vi "Build Table Results.vi"(11 "Table result references":T1) -> (3 "Table values":string[][](array[string]), 5 "Column headers":string[](array[string]))   [LabVIEW 2021, in "Single Tone_Audio DAC.lvlib"]
uses:
  Single Tone_Audio DAC.lvlib
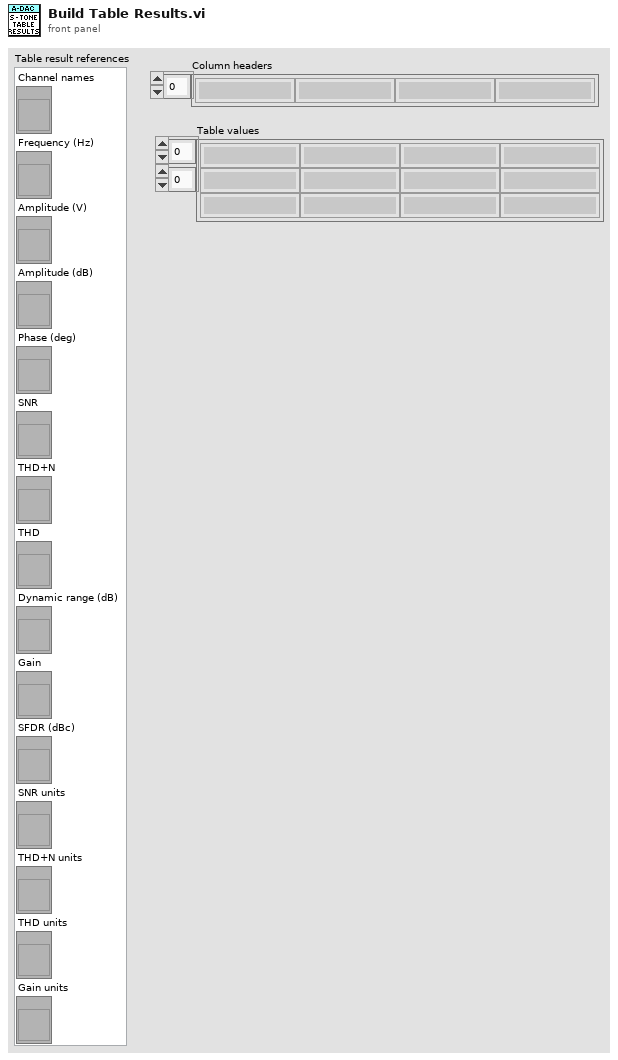
[diagram p1: front panel]
types:
  T1 = cluster{"Channel names":refnum<vi>, "Frequency (Hz)":refnum<vi>, "Amplitude (V)":refnum<vi>, "Amplitude (dB)":refnum<vi>, "Phase (deg)":refnum<vi>, "SNR":refnum<vi>, "THD+N":refnum<vi>, "THD":refnum<vi>, "Dynamic range (dB)":refnum<vi>, "Gain":refnum<vi>, "SFDR (dBc)":refnum<vi>, "SNR units":refnum<vi>, "THD+N units":refnum<vi>, "THD units":refnum<vi>, "Gain units":refnum<vi>}
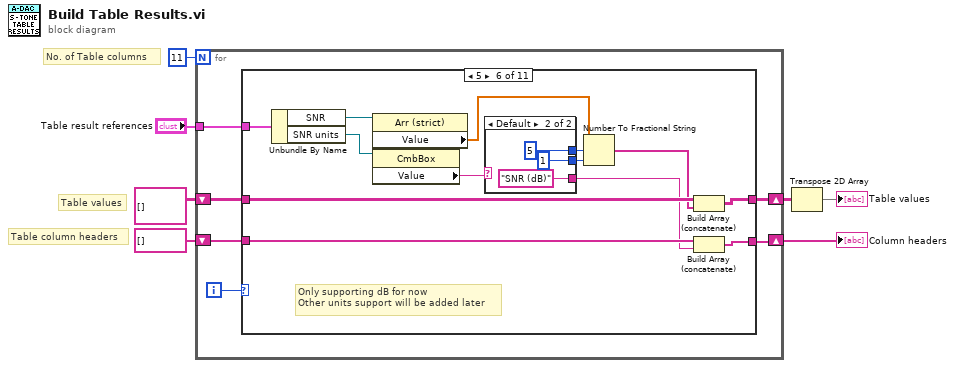
[diagram p0: block diagram]
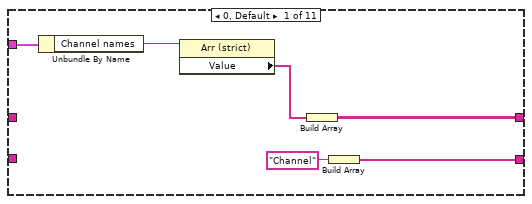
[diagram p2: hidden frame]
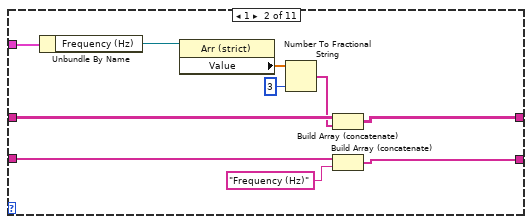
[diagram p3: hidden frame]
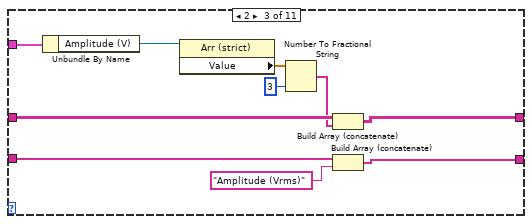
[diagram p4: hidden frame]
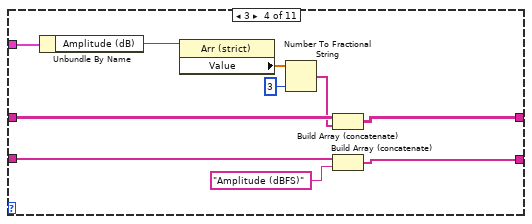
[diagram p5: hidden frame]
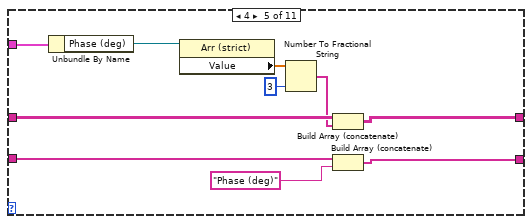
[diagram p6: hidden frame]
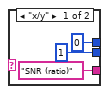
[diagram p7: hidden frame]
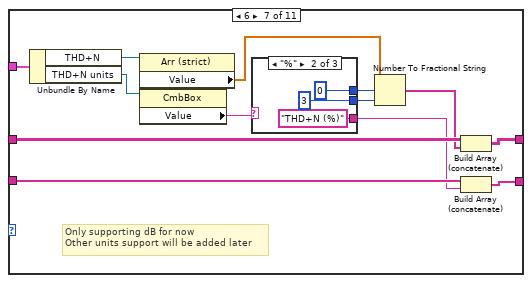
[diagram p8: hidden frame]
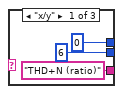
[diagram p9: hidden frame]
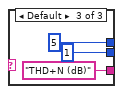
[diagram p10: hidden frame]
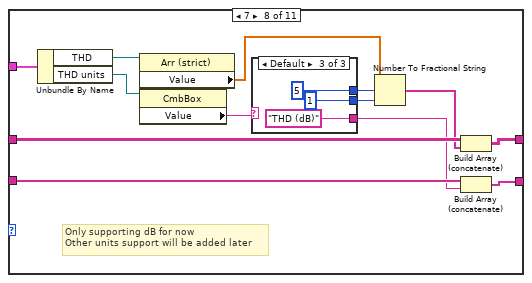
[diagram p11: hidden frame]
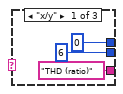
[diagram p12: hidden frame]
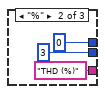
[diagram p13: hidden frame]
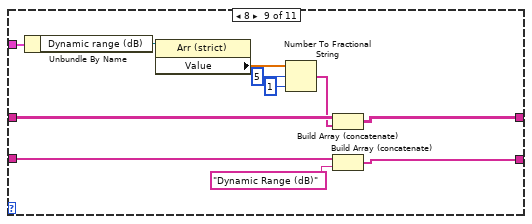
[diagram p14: hidden frame]
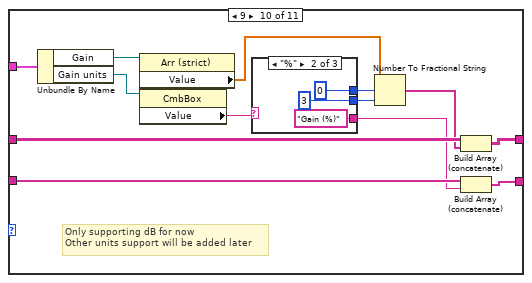
[diagram p15: hidden frame]
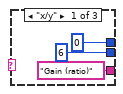
[diagram p16: hidden frame]
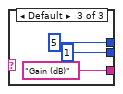
[diagram p17: hidden frame]
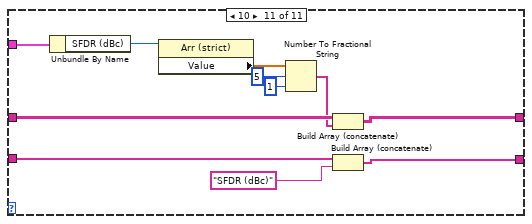
[diagram p18: hidden frame]
diagram:
  # "Table column headers"
  # "Table values"
  # "No. of Table columns"
  n1 = for {
    N: 11 -> [_]
    tunnel: "Table result references" -> [w12]
    shift-right: [w11] -> w3
    shift-left: string[][] [] -> [w10]
    shift-right: [w9] -> w2
    shift-left: string[] [] -> [w8]
    i -> [w13]
    n2 = case shown="5" w13 {
      tunnel: w12 -> [w19 w29 w39 w49 w59 w72 w91 w113 w133 w146 w166]
      tunnel: [w16 w22 w32 w42 w52 w66 w85 w107 w126 w140 w159] -> w11
      tunnel: w10 -> [_ w24 w34 w44 w54 w68 w87 w109 w128 w142 w161]
      tunnel: [w14 w20 w30 w40 w50 w64 w83 w105 w124 w138 w157] -> w9
      tunnel: w8 -> [_ w21 w31 w41 w51 w65 w84 w106 w125 w139 w158]
      frame 0, Default {
        n3 = Unbundle By Name(w19) -> ("Channel names"=w18:refnum<vi>)
        n4 = property class="Arr (strict)"(reference=w18) -> ("Value"=w17:string[])  [unwired: 1 in, 2 out]
        n5 = Build Array(w17) -> (w16:string[][])
        n6 = Build Array("Channel") -> (w14:string[])
      }
      frame 1 {
        n7 = Unbundle By Name(w29) -> ("Frequency (Hz)"=w28:refnum<vi>)
        n8 = property class="Arr (strict)"(reference=w28) -> ("Value"=w26:dbl[])  [unwired: 1 in, 2 out]
        n9 = Number To Fractional String(number=w26, precision (6)=i16 3) -> (F-format string=w23:string[])  [unwired: 2 in]
        n10 = Build Array (concatenate)(w24, w23) -> (w22:string[][])
        n11 = Build Array (concatenate)(w21, "Frequency (Hz)") -> (w20:string[])
      }
      frame 2 {
        n12 = Unbundle By Name(w39) -> ("Amplitude (V)"=w38:refnum<vi>)
        n13 = property class="Arr (strict)"(reference=w38) -> ("Value"=w36:dbl[])  [unwired: 1 in, 2 out]
        n14 = Number To Fractional String(number=w36, precision (6)=i16 3) -> (F-format string=w33:string[])  [unwired: 2 in]
        n15 = Build Array (concatenate)(w34, w33) -> (w32:string[][])
        n16 = Build Array (concatenate)(w31, "Amplitude (Vrms)") -> (w30:string[])
      }
      frame 3 {
        n17 = Unbundle By Name(w49) -> ("Amplitude (dB)"=w48:refnum<vi>)
        n18 = property class="Arr (strict)"(reference=w48) -> ("Value"=w46:dbl[])  [unwired: 1 in, 2 out]
        n19 = Number To Fractional String(number=w46, precision (6)=i16 3) -> (F-format string=w43:string[])  [unwired: 2 in]
        n20 = Build Array (concatenate)(w44, w43) -> (w42:string[][])
        n21 = Build Array (concatenate)(w41, "Amplitude (dBFS)") -> (w40:string[])
      }
      frame 4 {
        n22 = Unbundle By Name(w59) -> ("Phase (deg)"=w58:refnum<vi>)
        n23 = property class="Arr (strict)"(reference=w58) -> ("Value"=w56:dbl[])  [unwired: 1 in, 2 out]
        n24 = Number To Fractional String(number=w56, precision (6)=i16 3) -> (F-format string=w53:string[])  [unwired: 2 in]
        n25 = Build Array (concatenate)(w54, w53) -> (w52:string[][])
        n26 = Build Array (concatenate)(w51, "Phase (deg)") -> (w50:string[])
      }
      frame 5 {
        # "Only supporting dB for now\nOther units support will be added later"
        n27 = Unbundle By Name(w72) -> ("SNR"=w71:refnum<vi>, "SNR units"=w62:refnum<vi>)
        n28 = property class="Arr (strict)"(reference=w71) -> ("Value"=w70:dbl[])  [unwired: 1 in, 2 out]
        n29 = property class="CmbBox"(reference=w62) -> ("Value"=w61:string)  [unwired: 1 in, 2 out]
        n30 = case shown="Default" w61 {
          tunnel: [i16 1 ("precision (6)") i16 1 ("precision (6)")] -> w69
          tunnel: [i16 0 ("width (-)") i16 5 ("width (-)")] -> w63
          tunnel: ["SNR (ratio)" "SNR (dB)"] -> w60
          frame "x/y" {
          }
          frame Default {
          }
        }
        n31 = Number To Fractional String(number=w70, width (-)=w63, precision (6)=w69) -> (F-format string=w67:string[])  [unwired: 1 in]
        n32 = Build Array (concatenate)(w68, w67) -> (w66:string[][])
        n33 = Build Array (concatenate)(w65, w60) -> (w64:string[])
      }
      frame 6 {
        # "Only supporting dB for now\nOther units support will be added later"
        n34 = Unbundle By Name(w91) -> ("THD+N"=w90:refnum<vi>, "THD+N units"=w81:refnum<vi>)
        n35 = property class="Arr (strict)"(reference=w90) -> ("Value"=w89:dbl[])  [unwired: 1 in, 2 out]
        n36 = property class="CmbBox"(reference=w81) -> ("Value"=w80:string)  [unwired: 1 in, 2 out]
        n37 = case shown="\"%\"" w80 {
          tunnel: [i16 6 ("precision (6)") i16 3 ("precision (6)") i16 1 ("precision (6)")] -> w88
          tunnel: [i16 0 ("width (-)") i16 0 ("width (-)") i16 5 ("width (-)")] -> w82
          tunnel: ["THD+N (ratio)" "THD+N (%)" "THD+N (dB)"] -> w79
          frame "x/y" {
          }
          frame "%" {
          }
          frame Default {
          }
        }
        n38 = Number To Fractional String(number=w89, width (-)=w82, precision (6)=w88) -> (F-format string=w86:string[])  [unwired: 1 in]
        n39 = Build Array (concatenate)(w87, w86) -> (w85:string[][])
        n40 = Build Array (concatenate)(w84, w79) -> (w83:string[])
      }
      frame 7 {
        # "Only supporting dB for now\nOther units support will be added later"
        n41 = Unbundle By Name(w113) -> ("THD"=w112:refnum<vi>, "THD units"=w103:refnum<vi>)
        n42 = property class="Arr (strict)"(reference=w112) -> ("Value"=w111:dbl[])  [unwired: 1 in, 2 out]
        n43 = property class="CmbBox"(reference=w103) -> ("Value"=w102:string)  [unwired: 1 in, 2 out]
        n44 = case shown="Default" w102 {
          tunnel: [i16 6 ("precision (6)") i16 3 ("precision (6)") i16 1 ("precision (6)")] -> w110
          tunnel: [i16 0 ("width (-)") i16 0 ("width (-)") i16 5 ("width (-)")] -> w104
          tunnel: ["THD (ratio)" "THD (%)" "THD (dB)"] -> w101
          frame "x/y" {
          }
          frame "%" {
          }
          frame Default {
          }
        }
        n45 = Number To Fractional String(number=w111, width (-)=w104, precision (6)=w110) -> (F-format string=w108:string[])  [unwired: 1 in]
        n46 = Build Array (concatenate)(w109, w108) -> (w107:string[][])
        n47 = Build Array (concatenate)(w106, w101) -> (w105:string[])
      }
      frame 8 {
        n48 = Unbundle By Name(w133) -> ("Dynamic range (dB)"=w132:refnum<vi>)
        n49 = property class="Arr (strict)"(reference=w132) -> ("Value"=w130:dbl[])  [unwired: 1 in, 2 out]
        n50 = Number To Fractional String(number=w130, width (-)=i16 5, precision (6)=i16 1) -> (F-format string=w127:string[])  [unwired: 1 in]
        n51 = Build Array (concatenate)(w128, w127) -> (w126:string[][])
        n52 = Build Array (concatenate)(w125, "Dynamic Range (dB)") -> (w124:string[])
      }
      frame 9 {
        # "Only supporting dB for now\nOther units support will be added later"
        n53 = Unbundle By Name(w146) -> ("Gain"=w145:refnum<vi>, "Gain units"=w136:refnum<vi>)
        n54 = property class="Arr (strict)"(reference=w145) -> ("Value"=w144:dbl[])  [unwired: 1 in, 2 out]
        n55 = property class="CmbBox"(reference=w136) -> ("Value"=w135:string)  [unwired: 1 in, 2 out]
        n56 = case shown="\"%\"" w135 {
          tunnel: [i16 6 ("precision (6)") i16 3 ("precision (6)") i16 1 ("precision (6)")] -> w143
          tunnel: [i16 0 ("width (-)") i16 0 ("width (-)") i16 5 ("width (-)")] -> w137
          tunnel: ["Gain (ratio)" "Gain (%)" "Gain (dB)"] -> w134
          frame "x/y" {
          }
          frame "%" {
          }
          frame Default {
          }
        }
        n57 = Number To Fractional String(number=w144, width (-)=w137, precision (6)=w143) -> (F-format string=w141:string[])  [unwired: 1 in]
        n58 = Build Array (concatenate)(w142, w141) -> (w140:string[][])
        n59 = Build Array (concatenate)(w139, w134) -> (w138:string[])
      }
      frame 10 {
        n60 = Unbundle By Name(w166) -> ("SFDR (dBc)"=w165:refnum<vi>)
        n61 = property class="Arr (strict)"(reference=w165) -> ("Value"=w163:dbl[])  [unwired: 1 in, 2 out]
        n62 = Number To Fractional String(number=w163, width (-)=i16 5, precision (6)=i16 1) -> (F-format string=w160:string[])  [unwired: 1 in]
        n63 = Build Array (concatenate)(w161, w160) -> (w159:string[][])
        n64 = Build Array (concatenate)(w158, "SFDR (dBc)") -> (w157:string[])
      }
    }
  }
  "Column headers" <- w2
  n65 = Transpose 2D Array(2D array=w3) -> (transposed array=→"Table values":string[][])
